vi "CountHigh60.vi"(10 "60bit input":bool[](array[boolean])=[FALSE, FALSE, FALSE, FALSE, FALSE, FALSE, FALSE, FALSE, FALSE, FALSE, FALSE, FALSE, FALSE, FALSE, FALSE, FALSE, FALSE, FALSE, FALSE, FALSE, FALSE, FALSE, FALSE, FALSE, FALSE, FALSE, FALSE, FALSE, FALSE, FALSE, FALSE, FALSE, FALSE, FALSE, FALSE, FALSE, FALSE, FALSE, FALSE, FALSE, FALSE, FALSE, FALSE, FALSE, FALSE, FALSE, FALSE, FALSE, FALSE, FALSE, FALSE, FALSE, FALSE, FALSE, FALSE, FALSE, FALSE, FALSE, FALSE, FALSE], 11 "Previous high count":u16) -> (2 "New high count":u16)   [LabVIEW 2012]
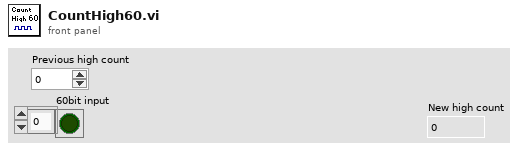
[diagram p1: front panel]
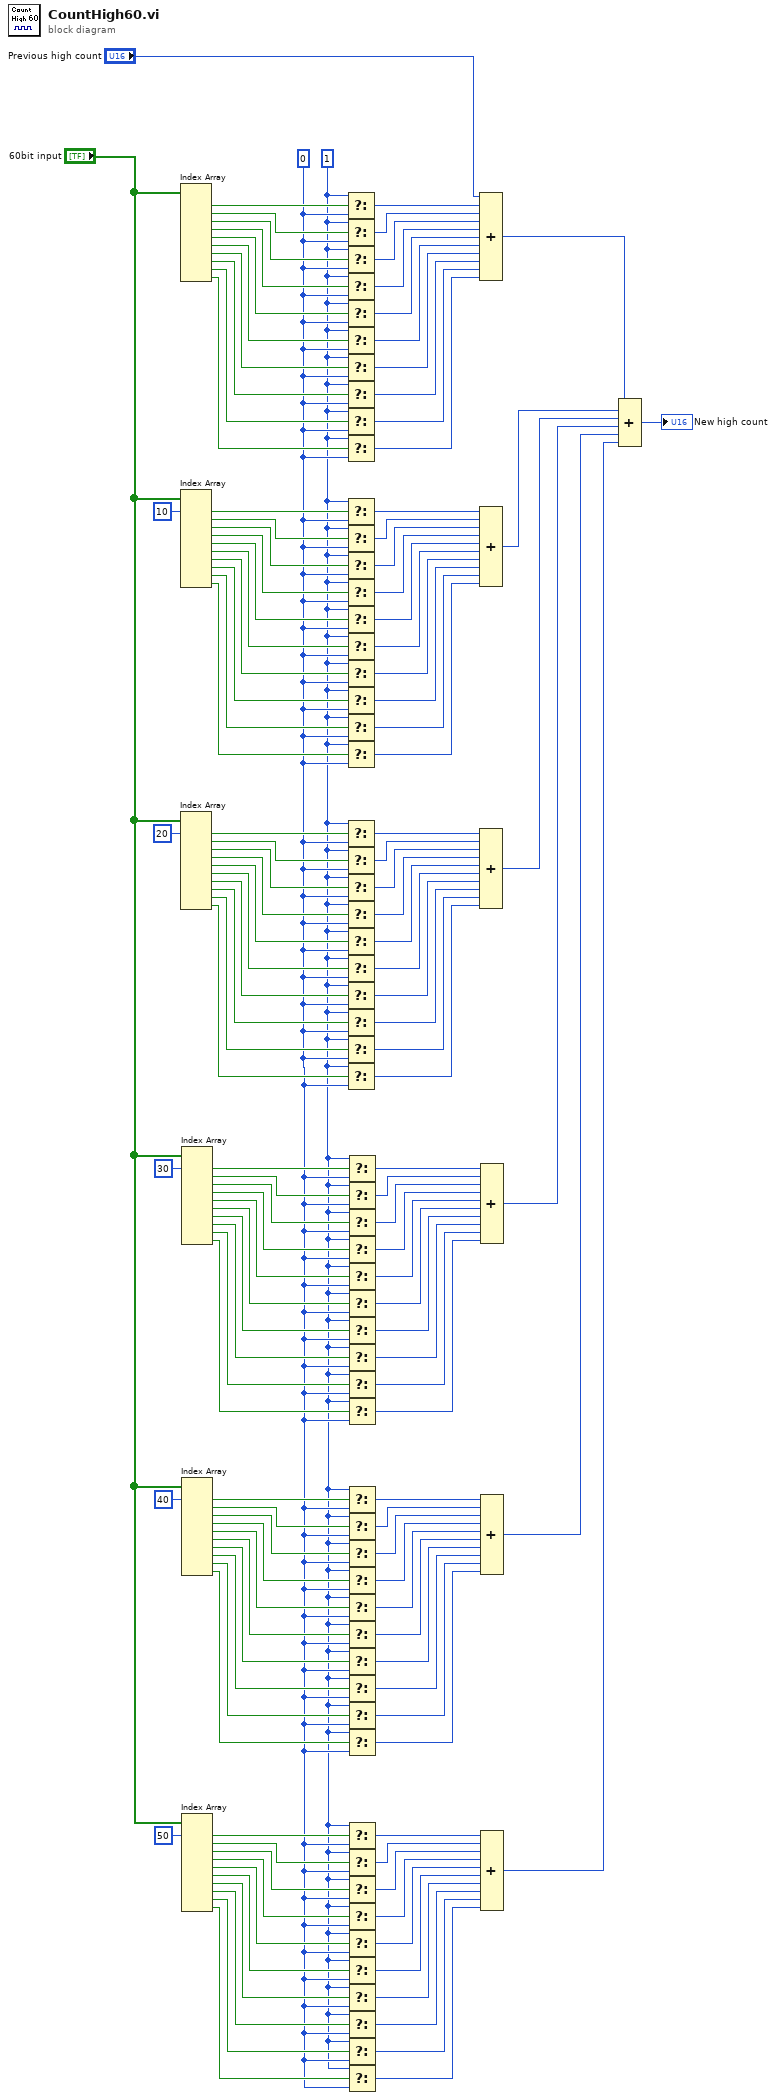
[diagram p0: block diagram]
diagram:
  w8 = u16 1
  w9 = u16 0
  n1 = Index Array(array="60bit input") -> (element #1=w136:bool, element #2=w135:bool, element #3=w134:bool, element #4=w133:bool, element #5=w132:bool, element #6=w131:bool, element #7=w130:bool, element #8=w129:bool, element #9=w128:bool, element #10=w127:bool)  [unwired: 10 in]
  n2 = Index Array(array="60bit input", index #1=10 ("index")) -> (element #1=w97:bool, element #2=w115:bool, element #3=w114:bool, element #4=w113:bool, element #5=w112:bool, element #6=w111:bool, element #7=w110:bool, element #8=w109:bool, element #9=w108:bool, element #10=w107:bool)  [unwired: 9 in]
  n3 = Index Array(array="60bit input", index #1=20 ("index")) -> (element #1=w76:bool, element #2=w94:bool, element #3=w93:bool, element #4=w92:bool, element #5=w91:bool, element #6=w90:bool, element #7=w89:bool, element #8=w88:bool, element #9=w87:bool, element #10=w86:bool)  [unwired: 9 in]
  n4 = Index Array(array="60bit input", index #1=30 ("index")) -> (element #1=w55:bool, element #2=w73:bool, element #3=w72:bool, element #4=w71:bool, element #5=w70:bool, element #6=w69:bool, element #7=w68:bool, element #8=w67:bool, element #9=w66:bool, element #10=w65:bool)  [unwired: 9 in]
  n5 = Index Array(array="60bit input", index #1=40 ("index")) -> (element #1=w34:bool, element #2=w52:bool, element #3=w51:bool, element #4=w50:bool, element #5=w49:bool, element #6=w48:bool, element #7=w47:bool, element #8=w46:bool, element #9=w45:bool, element #10=w44:bool)  [unwired: 9 in]
  n6 = Index Array(array="60bit input", index #1=50 ("index")) -> (element #1=w13:bool, element #2=w31:bool, element #3=w30:bool, element #4=w29:bool, element #5=w28:bool, element #6=w27:bool, element #7=w26:bool, element #8=w25:bool, element #9=w24:bool, element #10=w23:bool)  [unwired: 9 in]
  n7 = Select(t=w8, s=w136, f=w9) -> (s? t:f=w126:u16)
  n8 = Select(t=w8, s=w135, f=w9) -> (s? t:f=w125:u16)
  n9 = Select(t=w8, s=w134, f=w9) -> (s? t:f=w124:u16)
  n10 = Select(t=w8, s=w133, f=w9) -> (s? t:f=w123:u16)
  n11 = Select(t=w8, s=w132, f=w9) -> (s? t:f=w122:u16)
  n12 = Select(t=w8, s=w131, f=w9) -> (s? t:f=w121:u16)
  n13 = Select(t=w8, s=w130, f=w9) -> (s? t:f=w120:u16)
  n14 = Select(t=w8, s=w129, f=w9) -> (s? t:f=w119:u16)
  n15 = Select(t=w8, s=w128, f=w9) -> (s? t:f=w118:u16)
  n16 = Select(t=w8, s=w127, f=w9) -> (s? t:f=w117:u16)
  n17 = Select(t=w8, s=w97, f=w9) -> (s? t:f=w96:u16)
  n18 = Select(t=w8, s=w115, f=w9) -> (s? t:f=w106:u16)
  n19 = Select(t=w8, s=w114, f=w9) -> (s? t:f=w105:u16)
  n20 = Select(t=w8, s=w113, f=w9) -> (s? t:f=w104:u16)
  n21 = Select(t=w8, s=w112, f=w9) -> (s? t:f=w103:u16)
  n22 = Select(t=w8, s=w111, f=w9) -> (s? t:f=w102:u16)
  n23 = Select(t=w8, s=w110, f=w9) -> (s? t:f=w101:u16)
  n24 = Select(t=w8, s=w109, f=w9) -> (s? t:f=w100:u16)
  n25 = Select(t=w8, s=w108, f=w9) -> (s? t:f=w99:u16)
  n26 = Select(t=w8, s=w107, f=w9) -> (s? t:f=w98:u16)
  n27 = Select(t=w8, s=w76, f=w9) -> (s? t:f=w75:u16)
  n28 = Select(t=w8, s=w94, f=w9) -> (s? t:f=w85:u16)
  n29 = Select(t=w8, s=w93, f=w9) -> (s? t:f=w84:u16)
  n30 = Select(t=w8, s=w92, f=w9) -> (s? t:f=w83:u16)
  n31 = Select(t=w8, s=w91, f=w9) -> (s? t:f=w82:u16)
  n32 = Select(t=w8, s=w90, f=w9) -> (s? t:f=w81:u16)
  n33 = Select(t=w8, s=w89, f=w9) -> (s? t:f=w80:u16)
  n34 = Select(t=w8, s=w88, f=w9) -> (s? t:f=w79:u16)
  n35 = Select(t=w8, s=w87, f=w9) -> (s? t:f=w78:u16)
  n36 = Select(t=w8, s=w86, f=w9) -> (s? t:f=w77:u16)
  n37 = Select(t=w8, s=w55, f=w9) -> (s? t:f=w54:u16)
  n38 = Select(t=w8, s=w73, f=w9) -> (s? t:f=w64:u16)
  n39 = Select(t=w8, s=w72, f=w9) -> (s? t:f=w63:u16)
  n40 = Select(t=w8, s=w71, f=w9) -> (s? t:f=w62:u16)
  n41 = Select(t=w8, s=w70, f=w9) -> (s? t:f=w61:u16)
  n42 = Select(t=w8, s=w69, f=w9) -> (s? t:f=w60:u16)
  n43 = Select(t=w8, s=w68, f=w9) -> (s? t:f=w59:u16)
  n44 = Select(t=w8, s=w67, f=w9) -> (s? t:f=w58:u16)
  n45 = Select(t=w8, s=w66, f=w9) -> (s? t:f=w57:u16)
  n46 = Select(t=w8, s=w65, f=w9) -> (s? t:f=w56:u16)
  n47 = Select(t=w8, s=w34, f=w9) -> (s? t:f=w33:u16)
  n48 = Select(t=w8, s=w52, f=w9) -> (s? t:f=w43:u16)
  n49 = Select(t=w8, s=w51, f=w9) -> (s? t:f=w42:u16)
  n50 = Select(t=w8, s=w50, f=w9) -> (s? t:f=w41:u16)
  n51 = Select(t=w8, s=w49, f=w9) -> (s? t:f=w40:u16)
  n52 = Select(t=w8, s=w48, f=w9) -> (s? t:f=w39:u16)
  n53 = Select(t=w8, s=w47, f=w9) -> (s? t:f=w38:u16)
  n54 = Select(t=w8, s=w46, f=w9) -> (s? t:f=w37:u16)
  n55 = Select(t=w8, s=w45, f=w9) -> (s? t:f=w36:u16)
  n56 = Select(t=w8, s=w44, f=w9) -> (s? t:f=w35:u16)
  n57 = Select(t=w8, s=w13, f=w9) -> (s? t:f=w12:u16)
  n58 = Select(t=w8, s=w31, f=w9) -> (s? t:f=w22:u16)
  n59 = Select(t=w8, s=w30, f=w9) -> (s? t:f=w21:u16)
  n60 = Select(t=w8, s=w29, f=w9) -> (s? t:f=w20:u16)
  n61 = Select(t=w8, s=w28, f=w9) -> (s? t:f=w19:u16)
  n62 = Select(t=w8, s=w27, f=w9) -> (s? t:f=w18:u16)
  n63 = Select(t=w8, s=w26, f=w9) -> (s? t:f=w17:u16)
  n64 = Select(t=w8, s=w25, f=w9) -> (s? t:f=w16:u16)
  n65 = Select(t=w8, s=w24, f=w9) -> (s? t:f=w15:u16)
  n66 = Select(t=w8, s=w23, f=w9) -> (s? t:f=w14:u16)
  n67 = Compound Arithmetic op=ADD("Previous high count", w126, w125, w124, w123, w122, w121, w120, w119, w118, w117) -> (w7:u16)
  n68 = Compound Arithmetic op=ADD(w96, w106, w105, w104, w103, w102, w101, w100, w99, w98) -> (w5:u16)
  n69 = Compound Arithmetic op=ADD(w75, w85, w84, w83, w82, w81, w80, w79, w78, w77) -> (w4:u16)
  n70 = Compound Arithmetic op=ADD(w54, w64, w63, w62, w61, w60, w59, w58, w57, w56) -> (w3:u16)
  n71 = Compound Arithmetic op=ADD(w33, w43, w42, w41, w40, w39, w38, w37, w36, w35) -> (w2:u16)
  n72 = Compound Arithmetic op=ADD(w12, w22, w21, w20, w19, w18, w17, w16, w15, w14) -> (w1:u16)
  n73 = Compound Arithmetic op=ADD(w7, w5, w4, w3, w2, w1) -> (→"New high count":u16)
